vi "SetRelativePositionUm.vi"(8 "error in (no error)":errorcluster, 9 "RelativeMoveum":dbl min=0.0 max=200.0, 10 "Stage Label":string, 11 "Stage_MadCityLab in":refnum<class "Stage_MadCityLab.lvclass">) -> (0 "error out":errorcluster, 3 "Stage_MadCityLab out":refnum<class "Stage_MadCityLab.lvclass">)   [LabVIEW 2020, in "Stage_MadCityLab.lvlib" / "Stage_MadCityLab.lvclass"]
uses:
  Stage_MadCityLab.lvclass
  Stage_MadCityLab.lvclass/Stage_MadCityLab.ctl
  HAL Layer/Stage/Stage/Stage.lvclass
  Dependency/Madlib.dll
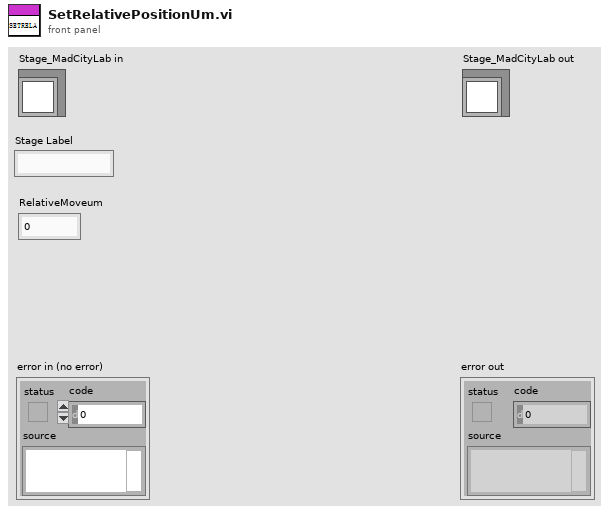
[diagram p1: front panel]
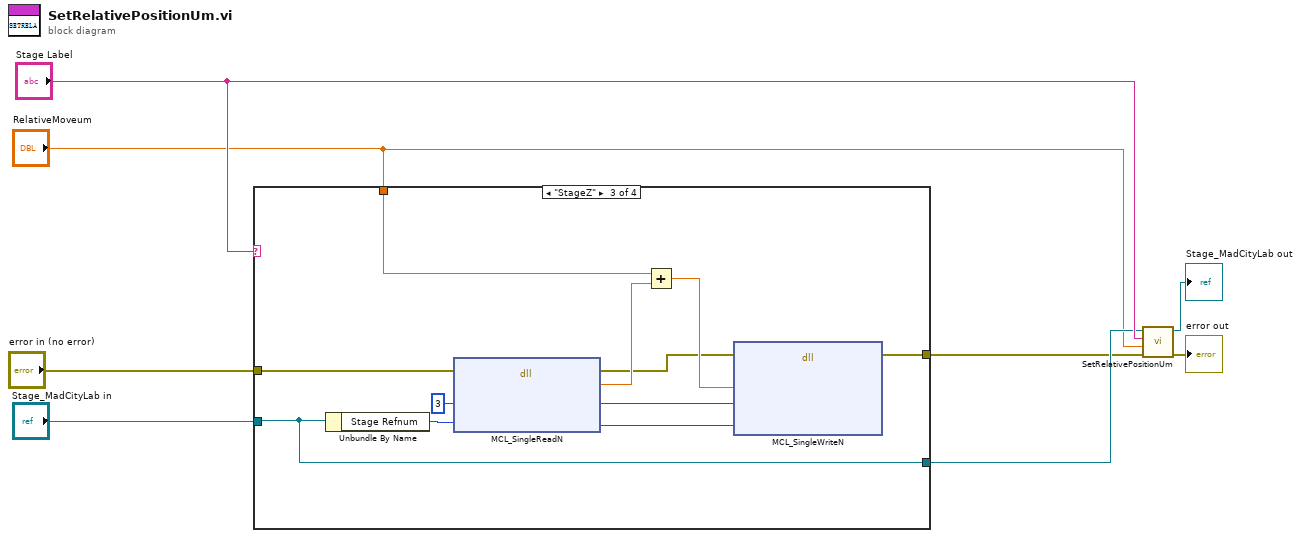
[diagram p0: block diagram]
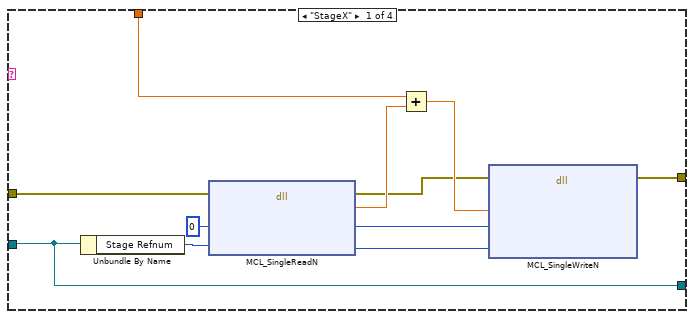
[diagram p2: hidden frame]
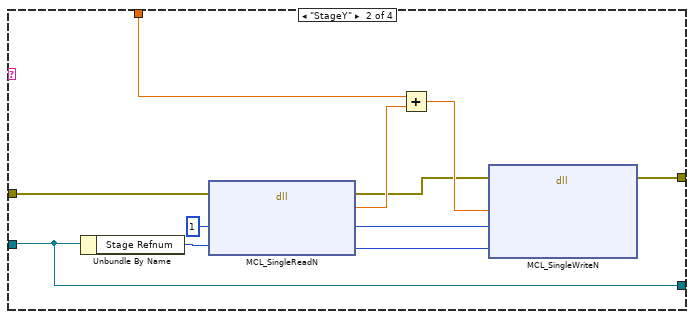
[diagram p3: hidden frame]
diagram:
  n1 = case shown="\"StageZ\"" "Stage Label" {
    tunnel: "Stage_MadCityLab in" -> [w9 w20 w31 w43]
    tunnel: [w9 w20 w31 w43] -> w4
    tunnel: "RelativeMoveum" -> [w13 w24 w35 _]
    tunnel: "error in (no error)" -> [w12 w23 w34 w42]
    tunnel: [w11 w22 w33 w42] -> w2
    frame "StageX" {
      n2 = Unbundle By Name(w9) -> ("Stage Refnum"=w14:i32)
      n3 = dll-call lib="E:/Development/DevHardSoftware/MMicroscopyAF/Model/Real Hardware/Stage_MadCityLab/Stage_MadCityLab/Dependency/Madlib.dll" fn="MCL_SingleReadN"(error in=w12, "axis"=u32 0, "handle"=w14) -> (error out=w15:errorcluster, "return type"=w17:dbl, "axis"=w18:u32, "handle"=w19:i32)  [unwired: 2 in, 1 out]
      n4 = Add(x=w13, y=w17) -> (x+y=w16:dbl)
      n5 = dll-call lib="E:/Development/DevHardSoftware/MMicroscopyAF/Model/Real Hardware/Stage_MadCityLab/Stage_MadCityLab/Dependency/Madlib.dll" fn="MCL_SingleWriteN"(error in=w15, "position"=w16, "axis"=w18, "handle"=w19) -> (error out=w11:errorcluster)  [unwired: 6 in, 1 out]
    }
    frame "StageY" {
      n6 = Unbundle By Name(w20) -> ("Stage Refnum"=w25:i32)
      n7 = dll-call lib="E:/Development/DevHardSoftware/MMicroscopyAF/Model/Real Hardware/Stage_MadCityLab/Stage_MadCityLab/Dependency/Madlib.dll" fn="MCL_SingleReadN"(error in=w23, "axis"=u32 1, "handle"=w25) -> (error out=w26:errorcluster, "return type"=w28:dbl, "axis"=w29:u32, "handle"=w30:i32)  [unwired: 2 in, 1 out]
      n8 = Add(x=w24, y=w28) -> (x+y=w27:dbl)
      n9 = dll-call lib="E:/Development/DevHardSoftware/MMicroscopyAF/Model/Real Hardware/Stage_MadCityLab/Stage_MadCityLab/Dependency/Madlib.dll" fn="MCL_SingleWriteN"(error in=w26, "position"=w27, "axis"=w29, "handle"=w30) -> (error out=w22:errorcluster)  [unwired: 6 in, 1 out]
    }
    frame "StageZ" {
      n10 = Unbundle By Name(w31) -> ("Stage Refnum"=w36:i32)
      n11 = dll-call lib="E:/Development/DevHardSoftware/MMicroscopyAF/Model/Real Hardware/Stage_MadCityLab/Stage_MadCityLab/Dependency/Madlib.dll" fn="MCL_SingleReadN"(error in=w34, "axis"=u32 3, "handle"=w36) -> (error out=w37:errorcluster, "return type"=w39:dbl, "axis"=w40:u32, "handle"=w41:i32)  [unwired: 2 in, 1 out]
      n12 = Add(x=w35, y=w39) -> (x+y=w38:dbl)
      n13 = dll-call lib="E:/Development/DevHardSoftware/MMicroscopyAF/Model/Real Hardware/Stage_MadCityLab/Stage_MadCityLab/Dependency/Madlib.dll" fn="MCL_SingleWriteN"(error in=w37, "position"=w38, "axis"=w40, "handle"=w41) -> (error out=w33:errorcluster)  [unwired: 6 in, 1 out]
    }
    frame Default {
    }
  }
  n14 = call-parent "SetRelativePositionUm.vi"("error in (no error)"=w2, "RelativeMoveum"="RelativeMoveum", "Stage Label"="Stage Label", "Stage in"=w4) -> ("error out"=→"error out":errorcluster, "Stage out"=→"Stage_MadCityLab out":refnum<class "Stage_MadCityLab.lvclass">)  [unwired: 6 in]
